vi "combination.vi"(0 "object in":refnum<class "212format_work.lvclass">, 1 "table输入":string(combo), 2 "仪器参数":string[](array[string]), 3 "簇":cluster{"QN":string, "MN":string, "PW":string}, 4 "参数":string, 5 "error in (no error)":errorcluster, 6 "仪器参数上传时间":enum16{"精确到小时", "原始时间"}(ring)) -> (14 "object out":refnum<class "212format_work.lvclass">, 18 "通讯包字符串":string, 19 "error out":errorcluster)   [LabVIEW 2016, in "212format_work.lvclass"]
uses:
  212format_work.lvclass
panel:
  in  "数据块":T1
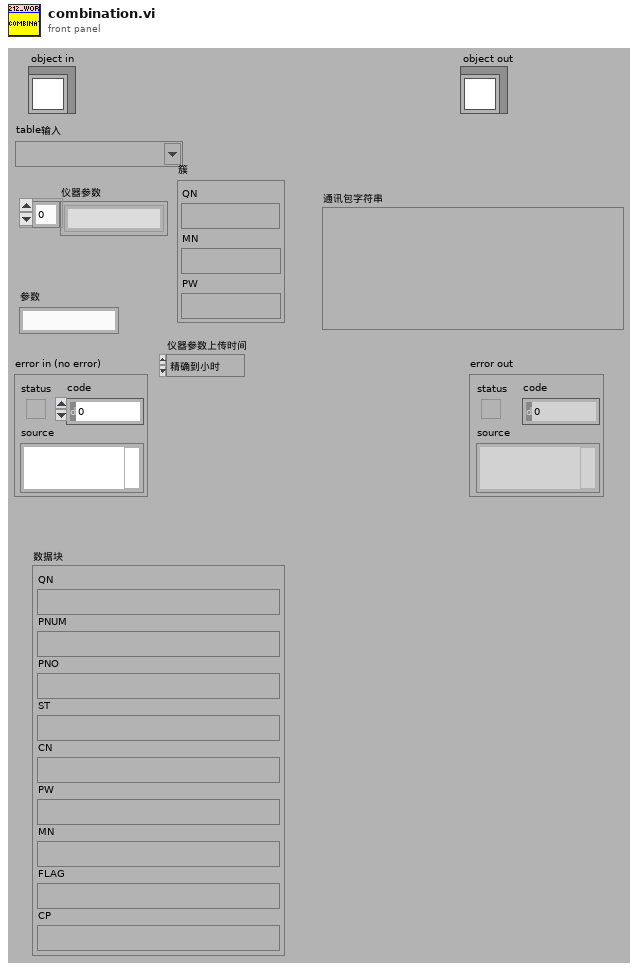
[diagram p1: front panel]
types:
  T1 = cluster{"QN":string, "ST":string, "CN":string, "PW":string, "MN":string, "FLAG":string, "PNUM":string, "PNO":string, "CP":string}
  T2 = typedef "212format_work.lvclass/interdata控件.ctl" = cluster{"数据发送协议":enum16{"2005-212协议", "2017-212协议"}, "枚举":enum16{"返回请求应答", "上传数据", "返回执行结果"}, "系统编码ST":string, "主动上报数据中":bool, "数据组合发送":bool, "地表水/污染源":bool, "应用环境":enum16{"STD", "GB212"}}
  T3 = typedef "212format_work.lvclass/data控件.ctl" = cluster{"选择发送的参数":string, "插值后的数组元素":cluster{"PH":string[][], "CODCr":string[][], "氨氮":string[][], "CODMn":string[][], "总氮":string[][], "总磷":string[][], "电导率":string[][], "水温":string[][], "DO":string[][], "浊度":string[][], "叶绿素":string[][], "藻密度":string[][], "铜":string[][], "盐度":string[][], "水位":string[][], "流速":string[][], "瞬时流量":string[][], "累积流量":string[][], "亚硝酸盐":string[][], "硫化物":string[][], "ORP":string[][], "铅":string[][], "镉":string[][], "锌":string[][], "镍":string[][], "锰":string[][], "汞":string[][], "气温":string[][], "气压":string[][], "风速":string[][], "风向":string[][], "盐度 2":string[][], "磷酸盐":string[][], "硝氮":string[][], "氟化物":string[][], "挥发酚":string[][], "氯化物":string[][]}, "register values":u16[], "columns输出":string[], "环境参数":string[][], "仪器编码":string, "实时数据发送间隔":u32, "实时数据参数":string, "参数系数簇":cluster{"CODMn":dbl, "CODCr":dbl, "DO":dbl, "铜":dbl, "PH":dbl, "氨氮":dbl, "比电导率":dbl, "水温":dbl, "COD":dbl, "浊度":dbl, "总氮":dbl, "总磷":dbl, "叶绿素a":dbl, "藻密度":dbl, "水位":dbl, "流速":dbl, "瞬时流量":dbl, "累积流量":dbl, "亚硝酸盐":dbl, "硫化物":dbl, "ORP":dbl, "铅":dbl, "镉":dbl, "锌":dbl, "镍":dbl, "锰":dbl, "汞":dbl, "气温":dbl, "气压":dbl, "风速":dbl, "风向":dbl, "盐度":dbl, "磷酸盐":dbl, "硝氮":dbl, "氟化物":dbl, "挥发酚":dbl, "氯化物":dbl}, "因子编码簇":cluster{"CODMn":string, "CODCr":string, "DO":string, "铜":string, "PH":string, "氨氮":string, "比电导率":string, "水温":string, "COD":string, "浊度":string, "总氮":string, "总磷":string, "叶绿素a":string, "藻密度":string, "水位":string, "流速":string, "瞬时流量":string, "累积流量":string, "亚硝酸盐":string, "硫化物":string, "ORP":string, "铅":string, "镉":string, "锌":string, "镍":string, "锰":string, "汞":string, "气温":string, "气压":string, "风速":string, "风向":string, "盐度":string, "磷酸盐":string, "硝氮":string, "氟化物":string, "挥发酚":string, "氯化物":string}, "小时数据发送次数":i32, "读取试剂余量的值":u16[], "参数编码":string, "数据数组大小":i32, "总包数":i32, "当前包号":i32, "columns":string[], "剖面多参数":string[][], "分包标准":i32}
  T4 = cluster{"PH":string[][], "CODCr":string[][], "氨氮":string[][], "CODMn":string[][], "总氮":string[][], "总磷":string[][], "电导率":string[][], "水温":string[][], "DO":string[][], "浊度":string[][], "叶绿素":string[][], "藻密度":string[][], "铜":string[][], "盐度":string[][], "水位":string[][], "流速":string[][], "瞬时流量":string[][], "累积流量":string[][], "亚硝酸盐":string[][], "硫化物":string[][], "ORP":string[][], "铅":string[][], "镉":string[][], "锌":string[][], "镍":string[][], "锰":string[][], "汞":string[][], "气温":string[][], "气压":string[][], "风速":string[][], "风向":string[][], "盐度 2":string[][], "磷酸盐":string[][], "硝氮":string[][], "氟化物":string[][], "挥发酚":string[][], "氯化物":string[][]}
  T5 = typedef "212format_work.lvclass/fkcommand控件.ctl" = cluster{"反控命令枚举":enum16{"返回请求应答", "返回执行结果"}, "执行结果定义":u16, "执行反馈":bool, "执行结果":u16, "是否判断反馈？":bool}
  T6 = cluster{"QN":string, "氯化物":string[][], "参数":string, "仪器参数":string[], "插值后的数组元素":cluster{"PH":string[][], "CODCr":string[][], "氨氮":string[][], "CODMn":string[][], "总氮":string[][], "总磷":string[][], "电导率":string[][], "水温":string[][], "DO":string[][], "浊度":string[][], "叶绿素":string[][], "藻密度":string[][], "铜":string[][], "盐度":string[][], "水位":string[][], "流速":string[][], "瞬时流量":string[][], "累积流量":string[][], "亚硝酸盐":string[][], "硫化物":string[][], "ORP":string[][], "铅":string[][], "镉":string[][], "锌":string[][], "镍":string[][], "锰":string[][], "汞":string[][], "气温":string[][], "气压":string[][], "风速":string[][], "风向":string[][], "盐度 2":string[][], "磷酸盐":string[][], "硝氮":string[][], "氟化物":string[][], "挥发酚":string[][], "氯化物":string[][]}}
  T7 = cluster{"cn":string, "flag":string, "cp":string, "qn":string, "PNUM":string, "PNO":string}
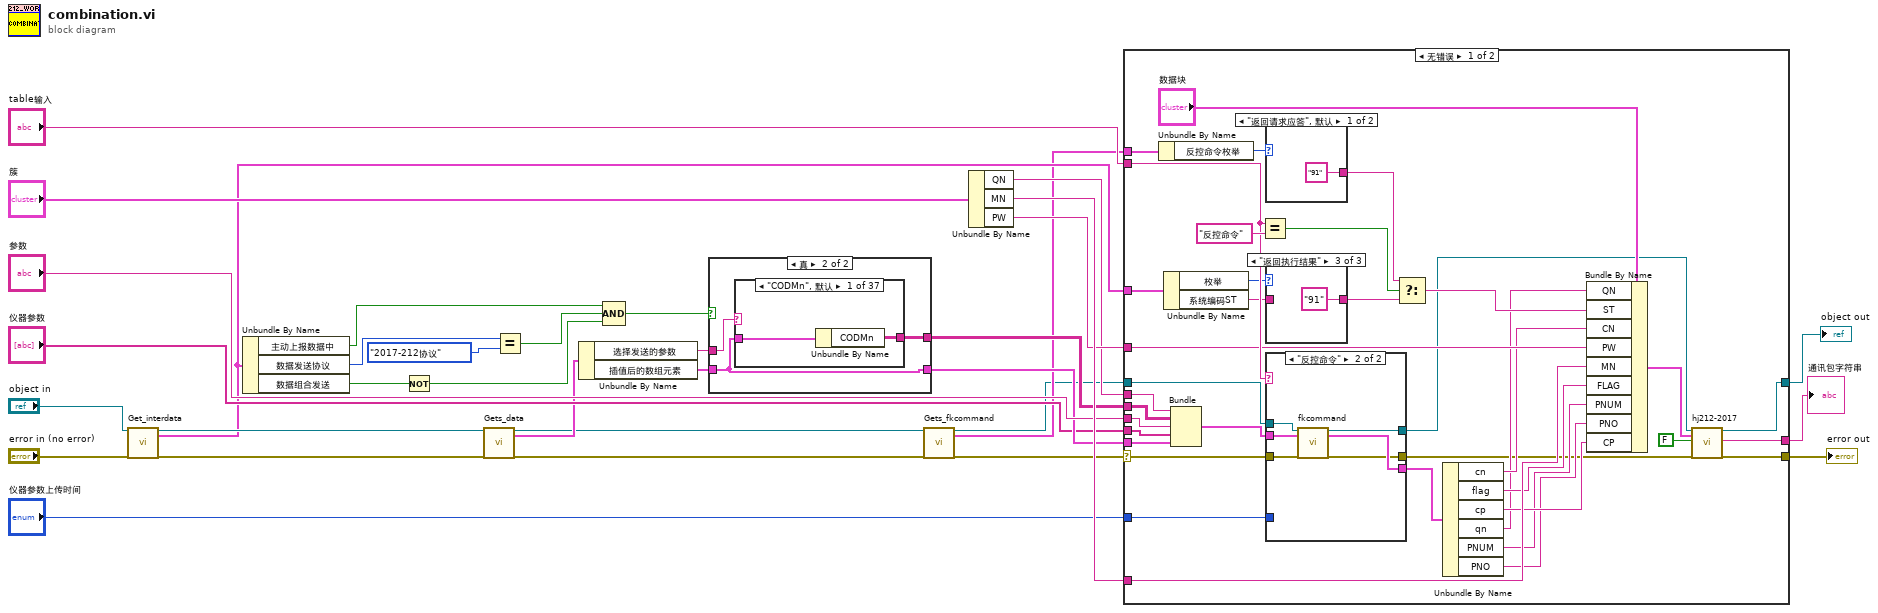
[diagram p0: block diagram]
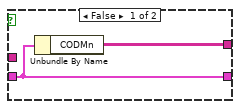
[diagram p2: hidden frame]
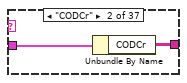
[diagram p3: hidden frame]
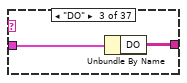
[diagram p4: hidden frame]
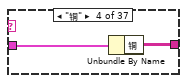
[diagram p5: hidden frame]
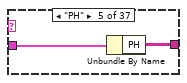
[diagram p6: hidden frame]
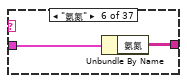
[diagram p7: hidden frame]
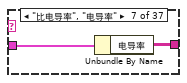
[diagram p8: hidden frame]
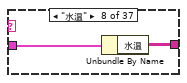
[diagram p9: hidden frame]
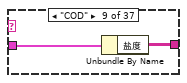
[diagram p10: hidden frame]
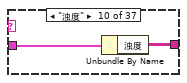
[diagram p11: hidden frame]
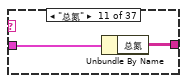
[diagram p12: hidden frame]
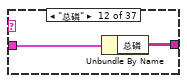
[diagram p13: hidden frame]
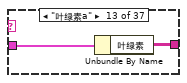
[diagram p14: hidden frame]
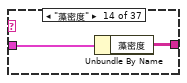
[diagram p15: hidden frame]
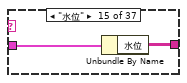
[diagram p16: hidden frame]
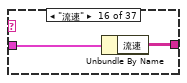
[diagram p17: hidden frame]
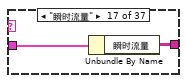
[diagram p18: hidden frame]
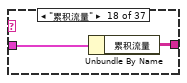
[diagram p19: hidden frame]
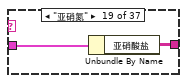
[diagram p20: hidden frame]
diagram:
  n1 = call-dynamic "Get_interdata.vi"("object in"="object in", "error in (no error)"="error in (no error)") -> ("object out"=w12:refnum<class "212format_work.lvclass">, "interdata"=w4:T2, "error out"=w7:errorcluster)  [unwired: 15 in]
  n2 = Unbundle By Name(w4) -> ("主动上报数据中"=w25:bool, "数据发送协议"=w24:enum16{"2005-212协议", "2017-212协议"}, "数据组合发送"=w21:bool)
  n3 = Not(x=w21) -> (.not. x?=w20:bool)
  n4 = call-dynamic "Gets_data.vi"("object in"=w12, "error in (no error)"=w7) -> ("object out"=w5:refnum<class "212format_work.lvclass">, "data"=w11:T3, "error out"=w6:errorcluster)  [unwired: 15 in]
  n5 = Equal?(x=w24, y=enum16{"2005-212协议", "2017-212协议"}."2017-212协议" ("数据发送版本")) -> (x = y?=w22:bool)
  n6 = Unbundle By Name(w11) -> ("选择发送的参数"=w10:string, "插值后的数组元素"=w9:T4)
  n7 = Compound Arithmetic op=AND ("复合运算")(w25, w22, w20) -> (w19:bool)
  n8 = case shown="真" w19 {
    tunnel: w10 -> [_ w38]
    tunnel: w9 -> [w35 w36]
    tunnel: [w35 w36] -> w16
    tunnel: [w34 w37] -> w15
    frame False {
      n9 = Unbundle By Name(w35) -> ("CODMn"=w34:string[][])
    }
    frame True {
      n10 = case shown="\"CODMn\", 默认" w38 {
        tunnel: [w39 w41 w43 w45 w47 w49 w51 w53 w55 w57 w59 w61 w63 w65 w67 w69 w71 w73 w75 w77 w79 w81 w83 w85 w87 w89 w91 w93 w95 w97 w99 w101 w103 w105 w107 w109 w111] -> w37
        tunnel: w36 -> [w40 w42 w44 w46 w48 w50 w52 w54 w56 w58 w60 w62 w64 w66 w68 w70 w72 w74 w76 w78 w80 w82 w84 w86 w88 w90 w92 w94 w96 w98 w100 w102 w104 w106 w108 w110 w112]
        frame "CODMn", Default {
          n11 = Unbundle By Name(w40) -> ("CODMn"=w39:string[][])
        }
        frame "CODCr" {
          n12 = Unbundle By Name(w42) -> ("CODCr"=w41:string[][])
        }
        frame "DO" {
          n13 = Unbundle By Name(w44) -> ("DO"=w43:string[][])
        }
        frame "铜" {
          n14 = Unbundle By Name(w46) -> ("铜"=w45:string[][])
        }
        frame "PH" {
          n15 = Unbundle By Name(w48) -> ("PH"=w47:string[][])
        }
        frame "氨氮" {
          n16 = Unbundle By Name(w50) -> ("氨氮"=w49:string[][])
        }
        frame "比电导率", "电导率" {
          n17 = Unbundle By Name(w52) -> ("电导率"=w51:string[][])
        }
        frame "水温" {
          n18 = Unbundle By Name(w54) -> ("水温"=w53:string[][])
        }
        frame "COD" {
          n19 = Unbundle By Name(w56) -> ("盐度"=w55:string[][])
        }
        frame "浊度" {
          n20 = Unbundle By Name(w58) -> ("浊度"=w57:string[][])
        }
        frame "总氮" {
          n21 = Unbundle By Name(w60) -> ("总氮"=w59:string[][])
        }
        frame "总磷" {
          n22 = Unbundle By Name(w62) -> ("总磷"=w61:string[][])
        }
        frame "叶绿素a" {
          n23 = Unbundle By Name(w64) -> ("叶绿素"=w63:string[][])
        }
        frame "藻密度" {
          n24 = Unbundle By Name(w66) -> ("藻密度"=w65:string[][])
        }
        frame "水位" {
          n25 = Unbundle By Name(w68) -> ("水位"=w67:string[][])
        }
        frame "流速" {
          n26 = Unbundle By Name(w70) -> ("流速"=w69:string[][])
        }
        frame "瞬时流量" {
          n27 = Unbundle By Name(w72) -> ("瞬时流量"=w71:string[][])
        }
        frame "累积流量" {
          n28 = Unbundle By Name(w74) -> ("累积流量"=w73:string[][])
        }
        frame "亚硝氮" {
          n29 = Unbundle By Name(w76) -> ("亚硝酸盐"=w75:string[][])
        }
        frame "硫化物" {
          n30 = Unbundle By Name(w78) -> ("硫化物"=w77:string[][])
        }
        frame "ORP" {
          n31 = Unbundle By Name(w80) -> ("ORP"=w79:string[][])
        }
        frame "铅" {
          n32 = Unbundle By Name(w82) -> ("铅"=w81:string[][])
        }
        frame "镉" {
          n33 = Unbundle By Name(w84) -> ("镉"=w83:string[][])
        }
        frame "锌" {
          n34 = Unbundle By Name(w86) -> ("锌"=w85:string[][])
        }
        frame "镍" {
          n35 = Unbundle By Name(w88) -> ("镍"=w87:string[][])
        }
        frame "锰" {
          n36 = Unbundle By Name(w90) -> ("锰"=w89:string[][])
        }
        frame "汞" {
          n37 = Unbundle By Name(w92) -> ("汞"=w91:string[][])
        }
        frame "气温" {
          n38 = Unbundle By Name(w94) -> ("气温"=w93:string[][])
        }
        frame "气压" {
          n39 = Unbundle By Name(w96) -> ("气压"=w95:string[][])
        }
        frame "风速" {
          n40 = Unbundle By Name(w98) -> ("风速"=w97:string[][])
        }
        frame "风向" {
          n41 = Unbundle By Name(w100) -> ("风向"=w99:string[][])
        }
        frame "盐度" {
          n42 = Unbundle By Name(w102) -> ("盐度 2"=w101:string[][])
        }
        frame "磷酸盐" {
          n43 = Unbundle By Name(w104) -> ("磷酸盐"=w103:string[][])
        }
        frame "硝氮" {
          n44 = Unbundle By Name(w106) -> ("硝氮"=w105:string[][])
        }
        frame "氟化物" {
          n45 = Unbundle By Name(w108) -> ("氟化物"=w107:string[][])
        }
        frame "挥发酚" {
          n46 = Unbundle By Name(w110) -> ("挥发酚"=w109:string[][])
        }
        frame "氯化物" {
          n47 = Unbundle By Name(w112) -> ("氯化物"=w111:string[][])
        }
      }
    }
  }
  n48 = call-dynamic "Gets_fkcommand.vi"("object in"=w5, "error in (no error)"=w6) -> ("object out"=w2:refnum<class "212format_work.lvclass">, "fkcommand"=w3:T5, "error out"=w1:errorcluster)  [unwired: 15 in]
  n49 = Unbundle By Name("簇") -> ("QN"=w26:string, "MN"=w28:string, "PW"=w27:string)
  n50 = case shown="无错误" w1 {
    selector: w1 -> [w126 w164]
    tunnel: [w125 w164] -> w33
    tunnel: [w147 w163] -> w32
    tunnel: w2 -> [w113 w163]
    tunnel: [w146 _] -> w30
    tunnel: "table输入" -> [w143 _]
    tunnel: w28 -> [w138 _]
    tunnel: w27 -> [w137 _]
    tunnel: w26 -> [w124 _]
    tunnel: "参数" -> [w122 _]
    tunnel: "仪器参数" -> [w121 _]
    tunnel: "仪器参数上传时间" -> [w128 _]
    tunnel: w16 -> [w120 _]
    tunnel: w15 -> [w123 _]
    tunnel: w4 -> [w118 _]
    tunnel: w3 -> [w117 _]
    frame No Error {
      n51 = Unbundle By Name(w117) -> ("反控命令枚举"=w115:enum16{"返回请求应答", "返回执行结果"})
      n52 = Unbundle By Name(w118) -> ("枚举"=w116:enum16{"返回请求应答", "上传数据", "返回执行结果"}, "系统编码ST"=w114:string)
      n53 = Bundle("QN"=w124, "氯化物"=w123, "参数"=w122, "仪器参数"=w121, "插值后的数组元素"=w120) -> (w119:T6)  [unwired: 1 in]
      n54 = Equal?(x=w143, y="反控命令") -> (x = y?=w142:bool)
      n55 = case shown="\"返回请求应答\", 默认" w115 {
        tunnel: ["91" "91"] -> w141
        frame "返回请求应答", Default {
        }
        frame "返回执行结果" {
        }
      }
      n56 = case shown="\"返回执行结果\"" w116 {
        tunnel: ["91" ("CN") w151 "91" ("CN")] -> w140
        tunnel: w114 -> [_ w151 _]
        frame "返回请求应答", Default {
        }
        frame "上传数据" {
        }
        frame "返回执行结果" {
        }
      }
      n57 = case shown="\"反控命令\"" w143 {
        tunnel: w113 -> [w156 w157]
        tunnel: [w156 w162] -> w136
        tunnel: [_ w161] -> w135
        tunnel: w128 -> [_ _]
        tunnel: [w155 w160] -> w127
        tunnel: w126 -> [w155 w159]
        tunnel: w119 -> [_ w158]
        frame "假", Default {
        }
        frame "反控命令" {
          n58 = call-dynamic "fkcommand.vi"("object in"=w157, "in"=w158, "error in (no error)"=w159) -> ("object out"=w162:refnum<class "212format_work.lvclass">, "out"=w161:T7, "error out"=w160:errorcluster)  [unwired: 14 in]
        }
      }
      n59 = Select(t=w141, s=w142, f=w140) -> (s? t:f=w139:string)
      n60 = Unbundle By Name(w135) -> ("cn"=w134:string, "flag"=w133:string, "cp"=w132:string, "qn"=w131:string, "PNUM"=w130:string, "PNO"=w129:string)
      n61 = Bundle By Name(cluster="数据块", "QN"=w131, "ST"=w139, "CN"=w134, "PW"=w137, "MN"=w138, "FLAG"=w133, "PNUM"=w130, "PNO"=w129, "CP"=w132) -> (w148:T1)
      n62 = call-dynamic "hj212-2017.vi"("object in"=w136, "数据段"=w148, "PWD？"=FALSE, "error in (no error)"=w127) -> ("object out"=w147:refnum<class "212format_work.lvclass">, "通讯包字符串"=w146:string, "error out"=w125:errorcluster)  [unwired: 12 in, 1 out]
    }
    frame Error {
    }
  }
  "error out" <- w33
  "object out" <- w32
  "通讯包字符串" <- w30
